vi "Draw Text (ARGB).vi"(4 "Thickness (Default: 1)":i32=1, 5 "Text Drawing Settings (Default: Simplex)":T1={"OpenCV Font Face"=enum."FONT_HERSHEY_SIMPLEX", "Font Scale"=1.0}, 6 "OpenCV Line Type (Default LINE_8)":T6=enum."LINE_8", 7 "ARGB Colour":T5={"Alpha"=255, "RGB"=0}, 8 "error in (no error)":errorcluster, 9 "Text":string, 10 "Origin":T3, 11 "ARGB Image":T4) -> (0 "error out":errorcluster, 3 "ARGB Image (Duplicate)":T4)   [LabVIEW 2020, in "g_ar_toolkit.image.lvlib"]
uses:
  g_ar_toolkit.image.lvlib
  Line Type.ctl
  ARGB Image.ctl
  ARGB Colour.ctl
  g_ar_toolkit.common/Image Point (Integer).ctl
  Text Drawing Settings.ctl
  Font Face.ctl
  0015c4fc-6a12-4f82-815b-6c2f827f408b.vi
  g_ar_toolkit.common/Module Path.vi
  <vilib>/Utility/error.llb/Error Cluster From Error Code.vi
  g_ar_toolkit.common/g_ar_toolkit.common.lvlib
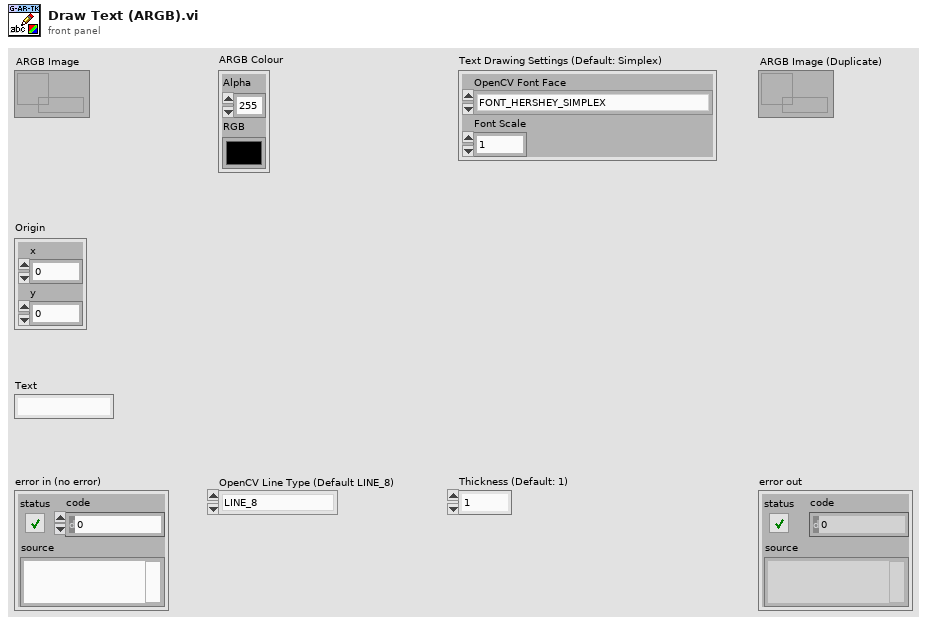
[diagram p1: front panel]
types:
  T1 = typedef "g_ar_toolkit.image.lvlib/Text Drawing Settings.ctl" = cluster{"OpenCV Font Face":T2, "Font Scale":dbl}
  T2 = typedef "g_ar_toolkit.image.lvlib/Font Face.ctl" = enum8{"FONT_HERSHEY_SIMPLEX", "FONT_HERSHEY_PLAIN", "FONT_HERSHEY_DUPLEX", "FONT_HERSHEY_COMPLEX", "FONT_HERSHEY_TRIPLEX", "FONT_HERSHEY_COMPLEX_SMALL", "FONT_HERSHEY_SCRIPT_SIMPLEX", "FONT_HERSHEY_SCRIPT_COMPLEX", "FONT_ITALIC"}
  T3 = typedef "g_ar_toolkit.common.lvlib/Image Point (Integer).ctl" = cluster{"x":i32, "y":i32}
  T4 = typedef "g_ar_toolkit.image.lvlib/ARGB Image.ctl" = refnum<data-value>
  T5 = typedef "g_ar_toolkit.image.lvlib/ARGB Colour.ctl" = cluster{"Alpha":u8, "RGB":u32}
  T6 = typedef "g_ar_toolkit.image.lvlib/Line Type.ctl" = enum8{"FILLED", "LINE_4", "LINE_8", "LINE_AA"}
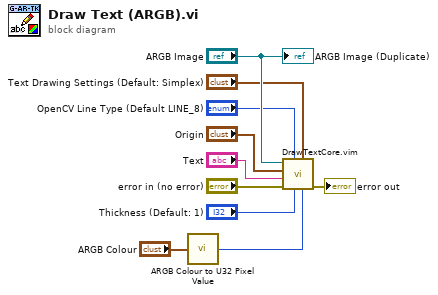
[diagram p0: block diagram]
diagram:
  n1 = call "ARGB Colour to U32 Pixel Value.vi"("ARGB Colour"="ARGB Colour") -> ("U32 Colour"=w2:u32)
  n2 = call "DrawTextCore.vim"("Colour"=w2, "Text Drawing Settings"="Text Drawing Settings (Default: Simplex)", "Thickness"="Thickness (Default: 1)", "OpenCV Line Type"="OpenCV Line Type (Default LINE_8)", "error in (no error)"="error in (no error)", "Text"="Text", "Origin"="Origin", "Src"="ARGB Image") -> ("error out"=→"error out":errorcluster)  [unwired: 3 in]
  "ARGB Image (Duplicate)" <- "ARGB Image"
